vi "TrashCan.vi"() -> ()   [LabVIEW 2020]
panel:
  out "Lid Status":string
  out "Clean Trash":bool
  out "Sonar Reading [Available Space]":dbl(graph)
  out "Space Available":bool
  in  "Table Control":string[][](table)
  in  "VISA resource name":refnum<visa-resource-name>
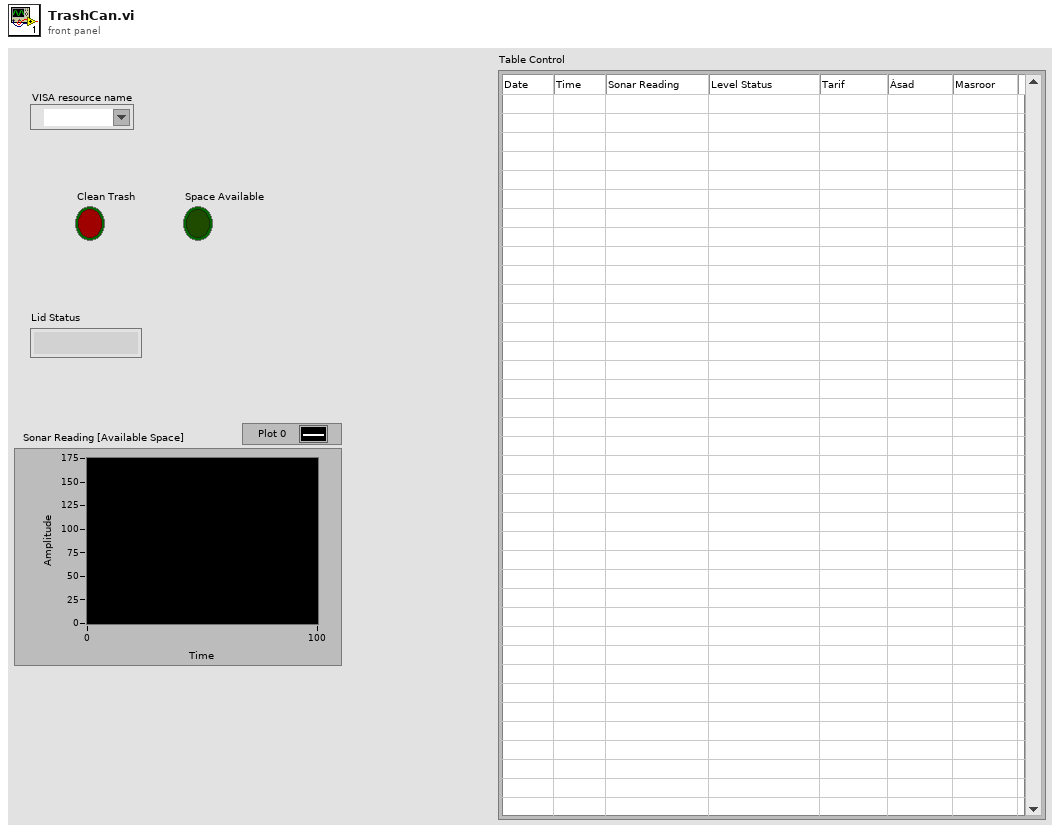
[diagram p1: front panel]
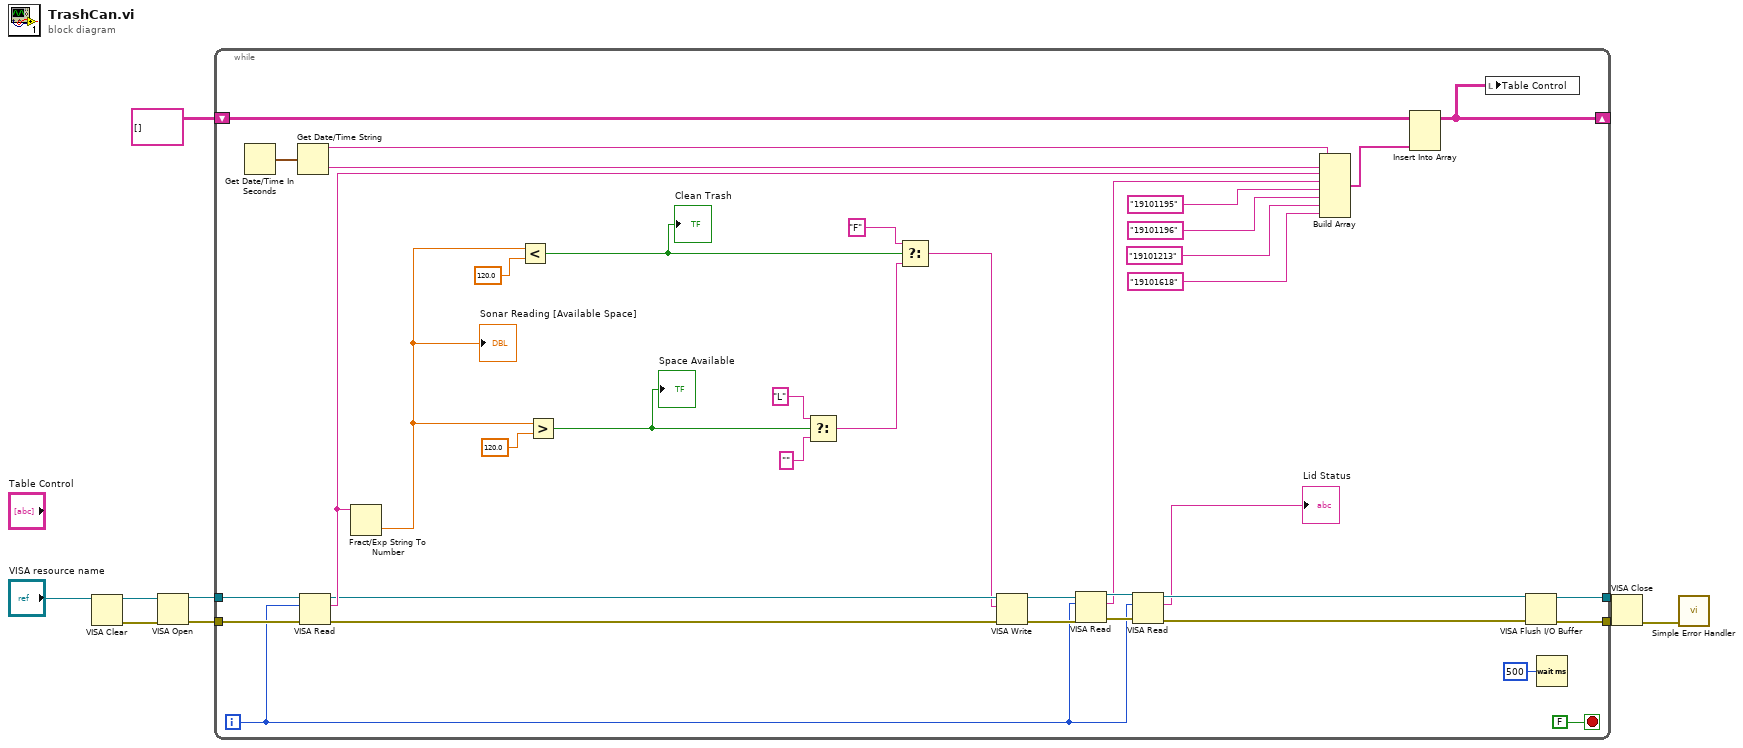
[diagram p0: block diagram]
diagram:
  n1 = VISA Clear(VISA resource name="VISA resource name") -> (VISA resource name out=w7:refnum<visa-resource-name>, error out=w6:errorcluster)  [unwired: 1 in]
  n2 = VISA Open(error in (no error)=w6, VISA resource name=w7) -> (VISA resource name=w9:refnum<visa-resource-name>, error out=w8:errorcluster)  [unwired: 3 in]
  n3 = while {
    tunnel: w9 -> [w47]
    tunnel: w8 -> [w46]
    tunnel: [w45] -> w5
    tunnel: [w44] -> w4
    shift-right: [w40] -> _
    shift-left: string[][] [] -> [w41]
    i -> [w22]
    stop <- FALSE stop-if-true
    n4 = Get Date/Time In Seconds() -> (seconds since 1Jan1904=w39:timestamp)
    n5 = Get Date/Time String(seconds (now)=w39) -> (date string=w38:string, time string=w37:string)  [unwired: 2 in]
    n6 = VISA Read(VISA resource name=w47, byte count=w22, error in (no error)=w46) -> (VISA resource name out=w31:refnum<visa-resource-name>, read buffer=w35:string, error out=w30:errorcluster)  [unwired: 1 out]
    n7 = Fract/Exp String To Number(string=w35) -> (number=w16:dbl)  [unwired: 3 in, 1 out]
    "Sonar Reading [Available Space]" <- w16
    n8 = Less?(x=w16, y=120.0) -> (x < y?=w15:bool)
    "Clean Trash" <- w15
    n9 = Greater?(x=w16, y=120.0) -> (0:w17:bool)
    "Space Available" <- w17
    n10 = Select(t="L", s=w17, f="") -> (s? t:f=w19:string)
    n11 = Select(t="F", s=w15, f=w19) -> (s? t:f=w18:string)
    n12 = VISA Write(VISA resource name=w31, write buffer=w18, error in (no error)=w30) -> (VISA resource name out=w29:refnum<visa-resource-name>, error out=w28:errorcluster)  [unwired: 1 out]
    n13 = VISA Read(VISA resource name=w29, byte count=w22, error in (no error)=w28) -> (VISA resource name out=w27:refnum<visa-resource-name>, read buffer=w25:string, error out=w26:errorcluster)  [unwired: 1 out]
    n14 = VISA Read(VISA resource name=w27, byte count=w22, error in (no error)=w26) -> (VISA resource name out=w24:refnum<visa-resource-name>, read buffer=→"Lid Status":string, error out=w23:errorcluster)  [unwired: 1 out]
    n15 = Build Array(w38, w37, w35, w25, "19101195", "19101196", "19101213", "19101618") -> (w36:string[])
    n16 = Insert Into Array(array=w41, new element=w36) -> (w40:string[][])  [unwired: 2 in]
    n17 = local write "Table Control"(w40) -> ()
    n18 = VISA Flush I/O Buffer(VISA resource name=w24, error in (no error)=w23) -> (VISA resource name out=w45:refnum<visa-resource-name>, error out=w44:errorcluster)  [unwired: 1 in]
    n19 = Wait (ms)(milliseconds to wait=u32 500) -> ()  [unwired: 1 out]
  }
  n20 = VISA Close(VISA resource name=w5, error in (no error)=w4) -> (error out=w3:errorcluster)
  n21 = call <vilib>:"Simple Error Handler.vi"("error in (no error)"=w3) -> ()  [unwired: 4 in, 5 out]
